vi "Plan Line, Continuous Acceleration.vi"(6 "Side":T3=enum."right", 7 "[6Tg]^-1":T1, 8 "queue":refnum<queue>, 9 "Joints":dbl[](array[numeric]), 11 "Goal":T2) -> (1 "Q size":i32)   [LabVIEW 2013]
uses:
  ROS/Code/SubVIs/BaxterSide.ctl
  Goal.ctl
  <vilib>/Analysis/Matrix/Datatypes/RealMatrix.ctl
  Fwd Kenimatics - array.vi
  <vilib>/Analysis/Matrix/Numeric/Multiply/Multiply - RM,RM.vi
  Baxter Examples/Arm Globals.vi
  <vilib>/Analysis/Matrix/NI_Matrix.lvlib
panel:
  in  "Stop":bool
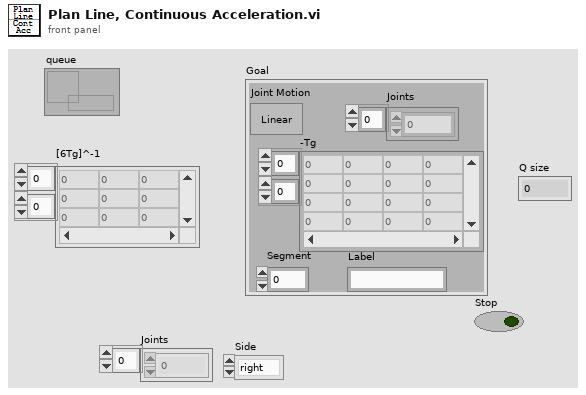
[diagram p1: front panel]
types:
  T1 = typedef "NI_Matrix.lvlib/RealMatrix.ctl" = dbl[][]
  T2 = typedef "Goal.ctl" = cluster{"Segment":dbl, "-Tg":T1, "Joints":dbl[], "Label":string, "Joint Motion":bool}
  T3 = typedef "BaxterSide.ctl" = enum16{"left", "right"}
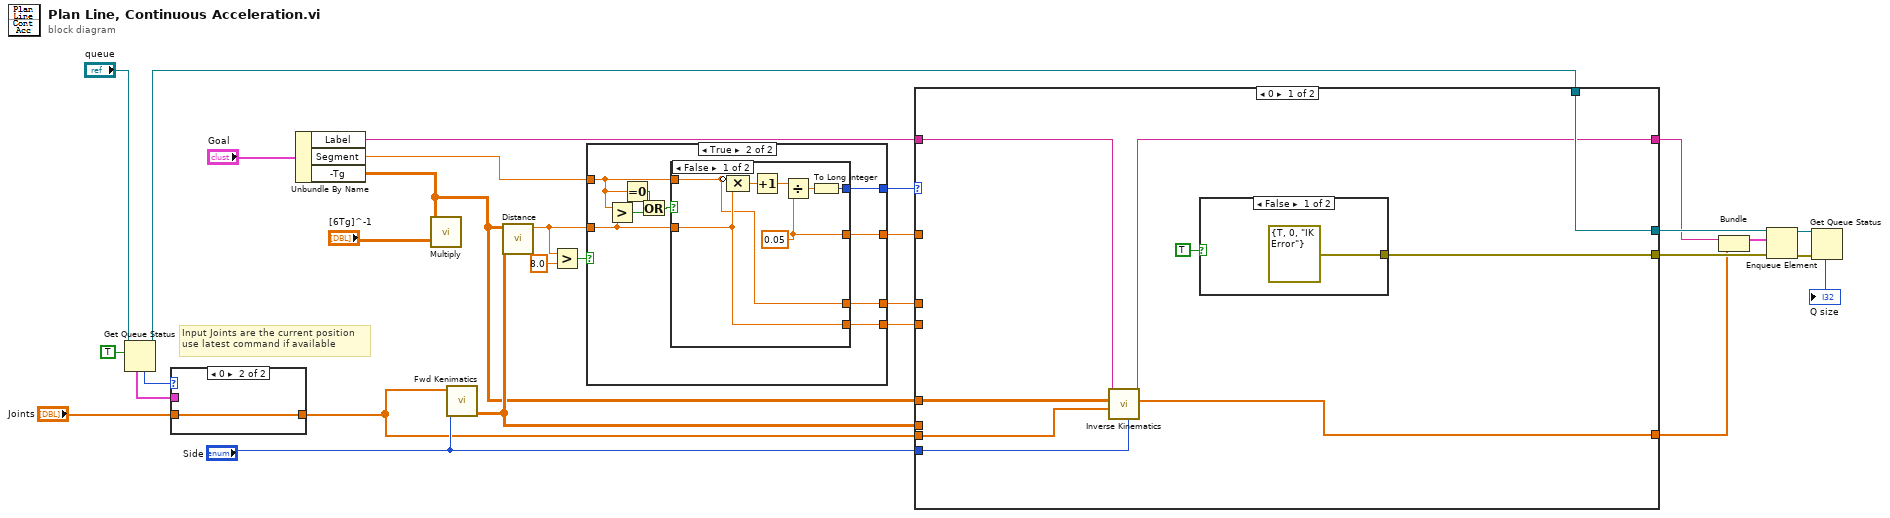
[diagram p0: block diagram]
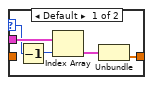
[diagram p2: hidden frame]
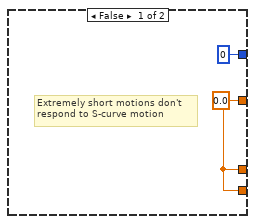
[diagram p3: hidden frame]
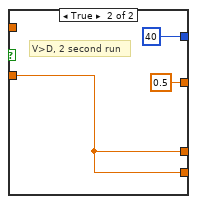
[diagram p4: hidden frame]
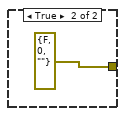
[diagram p5: hidden frame]
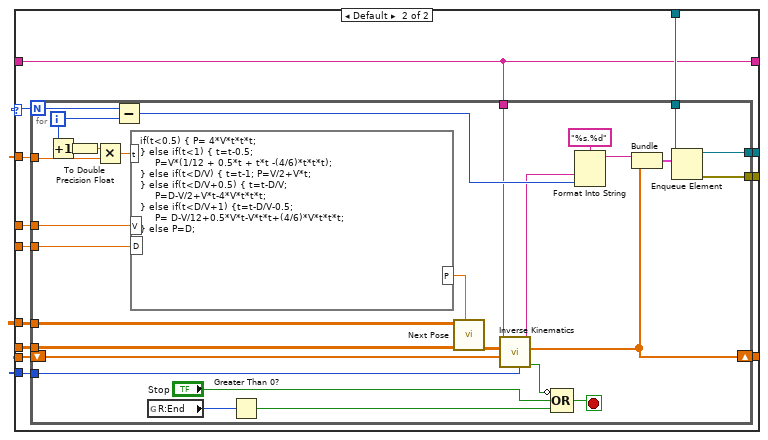
[diagram p6: hidden frame]
diagram:
  # "Input Joints are the current position\nuse latest command if available"
  n1 = Get Queue Status(queue="queue", return elements? (F)=TRUE) -> (queue out=w5:refnum<queue>, # elements in queue=w9:i32, elements=w7:cluster{string, "Joints":dbl[]}[])  [unwired: 1 in, 5 out]
  n2 = case shown="0" w9 {
    selector: w9 -> [w33 _]
    tunnel: w7 -> [w34 _]
    tunnel: [w30 w35] -> w3
    tunnel: "Joints" -> [_ w35]
    frame Default {
      n3 = Decrement(x=w33) -> (x-1=w32:i32)
      n4 = Index Array(array=w34, index=w32) -> (element=w31:cluster{string, "Joints":dbl[]})
      n5 = Unbundle(w31) -> ("Joints"=w30:dbl[])  [unwired: 1 out]
    }
    frame 0 {
    }
  }
  n6 = Unbundle By Name("Goal") -> ("Label"=w17:string, "Segment"=w13:dbl, "-Tg"=w1:T1)
  n7 = call-poly <vilib>:"Multiply.vi"("Real Matrix B"="[6Tg]^-1", "Real Matrix A"=w1) -> ()  [unwired: 1 out]
  n8 = call-poly "Fwd Kenimatics.vi"("Side"="Side", "Joints"=w3) -> ("Matrix"=w16:T1)  [unwired: 8 in, 1 out]
  n9 = call "Distance.vi"("Pose 2"=w16, "Pose 1"=w1) -> ("Distance"=w11:dbl)  [unwired: 9 in]
  n10 = Greater?(x=w11, y=8.0) -> (0:w12:bool)
  n11 = case shown="True" w12 {
    tunnel: [w36 w46] -> w27
    tunnel: [0 w45] -> w26
    tunnel: [w36 w44] -> w15
    tunnel: [w36 w43] -> w14
    tunnel: w11 -> [_ w42]
    tunnel: w13 -> [_ w39]
    frame False {
      w36 = 0.0 ("y")
      # "Extremely short motions don't\nrespond to S-curve motion"
    }
    frame True {
      n12 = Greater?(x=w39, y=w42) -> (0:w41:bool)
      n13 = Equal To 0?(x=w39) -> (x = 0?=w38:bool)
      n14 = Or(x=w38, y=w41) -> (x .or. y?=w40:bool)
      n15 = case shown="False" w40 {
        tunnel: w42 -> [w49 w55]
        tunnel: [w50 0.5 ("y")] -> w46
        tunnel: [w51 40] -> w45
        tunnel: w39 -> [w48 _]
        tunnel: [w48 w55] -> w44
        tunnel: [w49 w55] -> w43
        frame False {
          w50 = 0.05 ("y")
          n16 = Compound Arithmetic op=MULTIPLY(invert w48, w49) -> (w47:dbl)
          n17 = Increment(x=w47) -> (x+1=w53:dbl)
          n18 = Divide(x=w53, y=w50) -> (x/y=w52:dbl)
          n19 = To Long Integer(number=w52) -> (32bit integer=w51:i32)
        }
        frame True {
          # "V>D, 2 second run"
        }
      }
    }
  }
  n20 = case shown="0" w26 {
    selector: w26 -> [_ w72]
    tunnel: w27 -> [_ w80]
    tunnel: w5 -> [w65 w79]
    tunnel: "Side" -> [w60 w78]
    tunnel: w3 -> [w63 w77]
    tunnel: [w65 w76] -> w25
    tunnel: [w61 w75] -> w24
    tunnel: [w62 w74] -> w21
    tunnel: w1 -> [w64 w73]
    tunnel: w17 -> [w59 w71]
    tunnel: [w58 w71] -> w22
    tunnel: w16 -> [_ w70]
    tunnel: w15 -> [_ w69]
    tunnel: w14 -> [_ w68]
    frame 0 {
      n21 = call "Inverse Kinematics.vi"("Side"=w60, "Start"=w63, "Goal-matrix"=w64, "Label"=w59) -> ("J"=w62:dbl[], "Label"=w58:string)  [unwired: 4 in, 2 out]
      n22 = case shown="False" TRUE {
        tunnel: [errorcluster {"status"=TRUE, "code"=0, "source"="IK Error"} ("error out") errorcluster {"status"=FALSE, "code"=0, "source"=""} ("error out")] -> w61
        frame False {
        }
        frame True {
        }
      }
    }
    frame Default {
      n23 = for {
        N: w72 -> [w100]
        tunnel: w73 -> [w109]
        tunnel: w70 -> [w108]
        tunnel: w80 -> [w102]
        shift-right: [w97] -> w74
        shift-left: w77 -> [w104]
        tunnel: w79 -> [w107]
        tunnel: [w106] -> w76
        tunnel: [w105] -> w75
        tunnel: w78 -> [w87]
        tunnel: w71 -> [w86]
        tunnel: w69 -> [w91]
        tunnel: w68 -> [w90]
        i -> [w99]
        stop <- w96 stop-if-true
        n24 = Increment(x=w99) -> (x+1=w103:i32)
        n25 = To Double Precision Float(number=w103) -> (double precision float=w101:dbl)
        n26 = Multiply(x=w101, y=w102) -> (x*y=w92:dbl)
        n27 = Subtract(x=w100, y=w99) -> (x-y=w98:i32)
        n28 = formula code="if(t<0.5) { P= 4*V*t*t*t;\n} else if(t<1) { t=t-0.5; \n     P=V*(1/12 + 0.5*t + t*t -(4/6)*t*t*t);\n} else if(t<D/V) { t=t-1; P=V/2+V*t;\n} else if(t<D/V+0.5) { t=t-D/V;\n     P=D-V/2+V*t-4*V*t*t*t;\n} else if(t<D/V+1) {t=t-D/V-0.5;\n     P= D-V/12+0.5*V*t-V*t*t+(4/6)*V*t*t*t;\n} else P=D;"("t"=w92, "V"=w91, "D"=w90) -> ("P"=w89:dbl)
        n29 = global read "Arm Globals.vi" "R:End"() -> (w95:i32)
        n30 = Greater Than 0?(x=w95) -> (x > 0?=w81:bool)
        n31 = call "Next Pose.vi"("Step"=w89, "Last Pose"=w108, "Goal"=w109) -> ("Pose"=w94:T1)  [unwired: 7 in, 1 out]
        n32 = call "Inverse Kinematics.vi"("Side"=w87, "Start"=w104, "Goal-matrix"=w94, "Label"=w86) -> ("Found"=w88:bool, "J"=w97:dbl[], "Label"=w85:string)  [unwired: 4 in, 1 out]
        n33 = Compound Arithmetic op=OR(invert w88, "Stop", w81) -> (w96:bool)
        n34 = Format Into String(format string="%s.%d", w85, w98) -> (resulting string=w83:string)  [unwired: 2 in, 1 out]
        n35 = Bundle(w83, "J"=w97) -> (w82:cluster{string, "J":dbl[]})  [unwired: 1 in]
        n36 = Enqueue Element(queue=w107, element=w82) -> (queue out=w106:refnum<queue>, error out=w105:errorcluster)  [unwired: 2 in, 1 out]
      }
    }
  }
  n37 = Bundle("Label"=w22, "Joints"=w21) -> (w23:cluster{"Label":string, "Joints":dbl[]})  [unwired: 1 in]
  n38 = Enqueue Element(queue=w25, element=w23, error in (no error)=w24) -> (queue out=w20:refnum<queue>, error out=w19:errorcluster)  [unwired: 1 in, 1 out]
  n39 = Get Queue Status(queue=w20, error in (no error)=w19) -> (# elements in queue=→"Q size":i32)  [unwired: 1 in, 7 out]
